vi "Set Colors.vi"(8 "error in (no error)":errorcluster, 10 "Colors":u32[](array[colorbox]), 11 "Visualizer ID":T1) -> (0 "error out":errorcluster)   [LabVIEW 2017, in "Visualizer.lvlib"]
doc: "Set the colors to be used for waveforms plotted in the visualizer. The order of the colors in the input array corresponds to the order of waveforms pass into Set Waveforms.vi."
uses:
  Visualizer.lvlib
  Visualizer Type ID.ctl
  Message.ctl
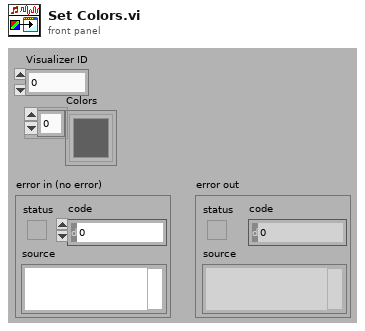
[diagram p1: front panel]
types:
  T1 = typedef "Visualizer.lvlib/Visualizer Type ID.ctl" = u32
  T2 = typedef "Visualizer.lvlib/Message.ctl" = cluster{"Command":string, "Data":variant}
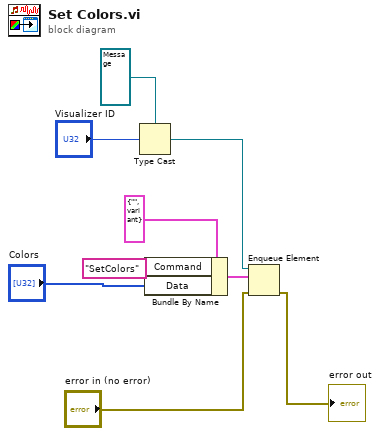
[diagram p0: block diagram]
diagram:
  n1 = Type Cast(type=refnum<queue> refnum ("queue out"), x="Visualizer ID") -> (*(type *) &x=w7:refnum<queue>)
  n2 = Bundle By Name(cluster=T2 {"Command"="", "Data"=variant} ("Message"), "Command"="SetColors", "Data"="Colors") -> (w1:T2)
  n3 = Enqueue Element(queue=w7, element=w1, error in (no error)="error in (no error)") -> (error out=→"error out":errorcluster)  [unwired: 1 in, 2 out]
